vi "VSI Open Device.vi"(9 "Reserved":i32, 10 "DevIndex":i32, 11 "DevType":i32) -> (3 "function return":i32)   [LabVIEW 2010, in "ControlSPI.lvlib"]
doc: "int WINAPI VSI_OpenDevice(int DevType,int DevIndex,int Reserved);"
uses:
  ControlSPI.lvlib
  ControlSPI/Ginkgo_Driver.dll
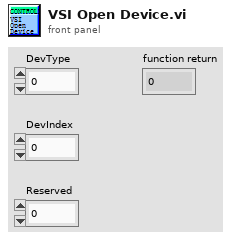
[diagram p1: front panel]
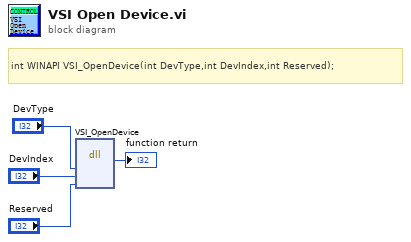
[diagram p0: block diagram]
diagram:
  # "int WINAPI VSI_OpenDevice(int DevType,int DevIndex,int Reserved);"
  n1 = dll-call lib="E:/Project/vt_ginkgo/truck/Ginkgo Driver/vs2010/Ginkgo_USB-I2C&SPI&CAN_API_v2.0.3.3/lib/labview_32bit/ControlSPI/Ginkgo_Driver.*" fn="VSI_OpenDevice"("DevType"="DevType", "DevIndex"="DevIndex", "Reserved"="Reserved") -> (→"function return":i32)  [unwired: 6 in, 2 out]
